vi "experiment control.vi"() -> ()   [LabVIEW 2012] (continued)
  T76 = cluster{"Wavemaster":cluster{"Serial Port":refnum<visa-resource-name>, "Wavelength":dbl, "Units":string, "VISA Name":refnum<visa-resource-name>, "Reading":bool, "Detected":bool}}
  T77 = cluster{"Header":cluster{"Element Names":string[], u8[]}, cluster{"Wavemaster":cluster{"Serial Port":refnum<visa-resource-name>, "Wavelength":dbl, "Units":string, "VISA Name":refnum<visa-resource-name>, "Reading":bool, "Detected":bool}}}
  T78 = cluster{"HP8341B":cluster{"GPIB Port":refnum<visa-resource-name>, "detected":bool, "rf":bool, "frequency":dbl, "stop frequency":dbl, "power":dbl, "sweep time":dbl, "Chirp":bool, "Pulse Modulate":bool, "Set frequency":dbl}}
  T79 = cluster{"Header":cluster{"Element Names":string[], u8[]}, cluster{"HP8341B":cluster{"GPIB Port":refnum<visa-resource-name>, "detected":bool, "rf":bool, "frequency":dbl, "stop frequency":dbl, "power":dbl, "sweep time":dbl, "Chirp":bool, "Pulse Modulate":bool, "Set frequency":dbl}}}
  T80 = cluster{"QuadDVM":cluster{"Serial Port":refnum<visa-resource-name>, "Quad DVM":dbl[][]}, "Magnetometer":cluster{"Active Boards":cluster{"Status":bool, "Board":string}[][], "USB ports":refnum<visa-resource-name>[], "Active Controllers":cluster{"Status":bool, "Number":dbl}[], "Measurements":cluster{"Bchip":dbl[][], "Status":dbl[], "Temperature":dbl, "Chip":dbl[], "Board":string, "Time":string}[]}, "Temperature Monitor":cluster{"measurements":cluster{"measurement":dbl, "location":string, "label":string}[], "last measurement time":string}}
  T81 = cluster{"Header":cluster{"Element Names":string[], u8[]}, cluster{"QuadDVM":cluster{"Serial Port":refnum<visa-resource-name>, "Quad DVM":dbl[][]}, "Magnetometer":cluster{"Active Boards":cluster{"Status":bool, "Board":string}[][], "USB ports":refnum<visa-resource-name>[], "Active Controllers":cluster{"Status":bool, "Number":dbl}[], "Measurements":cluster{"Bchip":dbl[][], "Status":dbl[], "Temperature":dbl, "Chip":dbl[], "Board":string, "Time":string}[]}, "Temperature Monitor":cluster{"measurements":cluster{"measurement":dbl, "location":string, "label":string}[], "last measurement time":string}}}
  T82 = cluster{"Frequency Counter":cluster{"GPIB Port":refnum<visa-resource-name>, "Frequency":dbl[]}}
  T83 = cluster{"Header":cluster{"Element Names":string[], u8[]}, cluster{"Frequency Counter":cluster{"GPIB Port":refnum<visa-resource-name>, "Frequency":dbl[]}}}
  T84 = cluster{"TDS5034B Oscilloscope":cluster{"GPIB Address":refnum<visa-resource-name>, "Detected":bool, "Channels":u16[], "Resolution":u16, "Frames":u16, "Trigger Position":dbl, "Trigger Level":dbl, "Measurements":cluster{"Type":string, "Value":dbl, "Source":string}[]}, "TDS2014 Oscilloscope":cluster{"GPIB Address":refnum<visa-resource-name>, "Detected":bool, "Channels":u16[], "Resolution":u16, "Frames":u16, "Trigger Position":dbl, "Trigger Level":dbl, "Measurements":cluster{"Type":string, "Value":dbl, "Source":string}[]}, "TDS5034B Data":cluster{"Y":dbl[], "t0":dbl, "dt":dbl}[], "TDS2014 Data":cluster{"Y":dbl[], "t0":dbl, "dt":dbl}[]}
  T85 = cluster{"Header":cluster{"Element Names":string[], u8[]}, cluster{"TDS5034B Oscilloscope":cluster{"GPIB Address":refnum<visa-resource-name>, "Detected":bool, "Channels":u16[], "Resolution":u16, "Frames":u16, "Trigger Position":dbl, "Trigger Level":dbl, "Measurements":cluster{"Type":string, "Value":dbl, "Source":string}[]}, "TDS2014 Oscilloscope":cluster{"GPIB Address":refnum<visa-resource-name>, "Detected":bool, "Channels":u16[], "Resolution":u16, "Frames":u16, "Trigger Position":dbl, "Trigger Level":dbl, "Measurements":cluster{"Type":string, "Value":dbl, "Source":string}[]}, "TDS5034B Data":cluster{"Y":dbl[], "t0":dbl, "dt":dbl}[], "TDS2014 Data":cluster{"Y":dbl[], "t0":dbl, "dt":dbl}[]}}
  T86 = cluster{"Trap Agilent":cluster{"USB":refnum<visa-resource-name>, "Amplitude":dbl, "Frequency":dbl, "Phase":dbl, "Upload":bool, "Output":bool}}
  T87 = cluster{"Header":cluster{"Element Names":string[], u8[]}, cluster{"Trap Agilent":cluster{"USB":refnum<visa-resource-name>, "Amplitude":dbl, "Frequency":dbl, "Phase":dbl, "Upload":bool, "Output":bool}}}
  T88 = cluster{"Jessica":T17, "Bertha":cluster{"wavelength":dbl, "locked":bool, "DIO64":string, "scan start":dbl, "scan end":dbl, "progress":u8, "scan step":dbl, "scan":bool, "setpoint":dbl, "wavelengths":dbl[]}, "Cora":cluster{"wavelength":dbl, "locked":bool, "DIO64":string, "scan start":dbl, "scan end":dbl, "progress":u8, "scan step":dbl, "scan":bool, "setpoint":dbl}, "Stella":cluster{"wavelength":dbl, "locked":bool, "lock tolerance":dbl, "setpoint":dbl, "scan start":dbl, "scan end":dbl, "progress":u8, "scan step":dbl, "scan":bool, "AI Channel":tag}, "Toptica":cluster{"wavelength":dbl, "locked":bool, "scan start":dbl, "scan end":dbl, "progress":u8, "scan step":dbl, "scan":bool, "AI Channel":tag}}
  T89 = cluster{"Header":cluster{"Element Names":string[], u8[]}, cluster{"Jessica":T17, "Bertha":cluster{"wavelength":dbl, "locked":bool, "DIO64":string, "scan start":dbl, "scan end":dbl, "progress":u8, "scan step":dbl, "scan":bool, "setpoint":dbl, "wavelengths":dbl[]}, "Cora":cluster{"wavelength":dbl, "locked":bool, "DIO64":string, "scan start":dbl, "scan end":dbl, "progress":u8, "scan step":dbl, "scan":bool, "setpoint":dbl}, "Stella":cluster{"wavelength":dbl, "locked":bool, "lock tolerance":dbl, "setpoint":dbl, "scan start":dbl, "scan end":dbl, "progress":u8, "scan step":dbl, "scan":bool, "AI Channel":tag}, "Toptica":cluster{"wavelength":dbl, "locked":bool, "scan start":dbl, "scan end":dbl, "progress":u8, "scan step":dbl, "scan":bool, "AI Channel":tag}}}
  T90 = cluster{"Header":cluster{"Element Names":string[], u8[]}, cluster{"Date":string, "Time":string}}
  T91 = cluster{"Switch Scan[0]":bool, "Switch Scan[1]":bool, "Switch Scan[2]":bool, "Switch Scan[3]":bool, "Switch Scan[4]":bool}
  T92 = cluster{"upper":dbl, "lower":dbl, "DurationUpper":dbl, "DurationLower":dbl, "Upper T":dbl, "Lower T":dbl}
  T93 = cluster{"Task":string, "begin time":dbl, "begin edge":bool, "begin reference":string, "end time":dbl, "end edge":bool, "end reference":string, "Chops":bool[]}
  T94 = cluster{"Down":cluster{"Frequency":dbl, "Phase":dbl, "Amplitude":dbl}[], "Up":cluster{"Frequency":dbl, "Phase":dbl, "Amplitude":dbl}[]}
  T95 = cluster{"Frequency":dbl, "Phase":dbl, "Amplitude":dbl}[]
  T96 = cluster{"Frequency":dbl, "Phase":dbl, "Duty Cycle":dbl, "Trigger":bool}[]
  T97 = cluster{"Frequency":dbl, "Phase":dbl, "Duty Cycle":dbl, "Trigger":bool}
  T98 = cluster{"variable":string, "scan string":string, "randomize":bool, "enable":bool}
  T99 = cluster{"Task":string, "Reference":string, "Begin":dbl, "Chops 2":bool[]}
  T100 = cluster{"Frequency":dbl, "Phase":dbl, "Amplitude":dbl}
  T101 = typedef "cw_template.ctl" = cluster{"wavelength":dbl, "name":string, "setpoint":dbl, "enable":bool, "lock":bool, "Priority":u8, "P":u8, "I":u8, "D":u8, "reset":bool, "analog channel":tag, "voltage":dbl, "exposure":u16, "range":dbl}
  T102 = typedef "pulse_template.ctl" = cluster{"wavelength":dbl, "name":string, "digital channel":tag}
  T103 = cluster{"Channel":string, "Name":string, "plot":bool}[]
  T104 = cluster{"system clock offset":bool, "system clock offset":bool, "open":bool, "open":bool, "multidevice sync mask":bool, "multidevice sync status":bool, "sync master enable":bool, "auto sync enable":bool, "open":bool, "open":bool, "open":bool, "open":bool, "all channel clear phase accumulator":bool, "all channel autoclear phase accumulator":bool, "all channel clear sweep accumulator":bool, "all channel autoclear sweep accumulator":bool}
  T105 = cluster{"Begin (ms)":dbl, "Begin (ms)":dbl, "DIO64 Line 1":bool[], "DIO64 Line 2":bool[], "DIO64 Line 3":bool[], "DIO64 Line 4":bool[]}
  T106 = cluster{"Begin (ms)":dbl, "Begin (ms)":dbl, "DIO64 Line 1":bool[], "DIO64 Line 2":bool[], "DIO64 Line 3":bool[], "DIO64 Line 4":bool[]}[]
  T107 = cluster{"Begin (ms)":dbl, "Begin (ms)":dbl, "DIO64 Line 4":bool[], "DIO64 Line 4":bool[], "DIO64 Line 4":bool[], "DIO64 Line 4":bool[]}
  T108 = cluster{"Begin (ms)":dbl, "Begin (ms)":dbl, "DIO64 Line 4":bool[], "DIO64 Line 4":bool[], "DIO64 Line 4":bool[], "DIO64 Line 4":bool[]}[]
  T109 = cluster{"Type":string, "Value":dbl, "Source":string}[]
  T110 = cluster{"Type":string, "Value":dbl, "Source":string}
  T111 = typedef "LVStringsAndValuesArrayTypeDef_U16.ctl" = cluster{"String":string, "Value":u16}[]
  T112 = typedef "LVRangeTypeDef.ctl" = cluster{"Minimum":dbl, "Maximum":dbl, "Increment":dbl, "Minor Increment":dbl, "Start":dbl}
  T113 = cluster{"start":dbl, "end":dbl, "ramp time":u8, "edge":bool}[]
  T114 = cluster{"Bchip":dbl[][], "Status":dbl[], "Temperature":dbl, "Chip":dbl[], "Board":string, "Time":string}[]
  T115 = cluster{"error":bool, "code":i32, "source":string}
  T116 = typedef "LVSelectionTypeDef.ctl" = cluster{"Selection Start":u32, "Selection End":u32}
  T117 = cluster{"32bit integer":i32, "32bit integer":u16}
  T118 = cluster{"Name":string, "DIO64 Line 1":bool[], "DIO64 Line 2":bool[], "DIO64 Line 3":bool[], "DIO64 Line 4":bool[]}
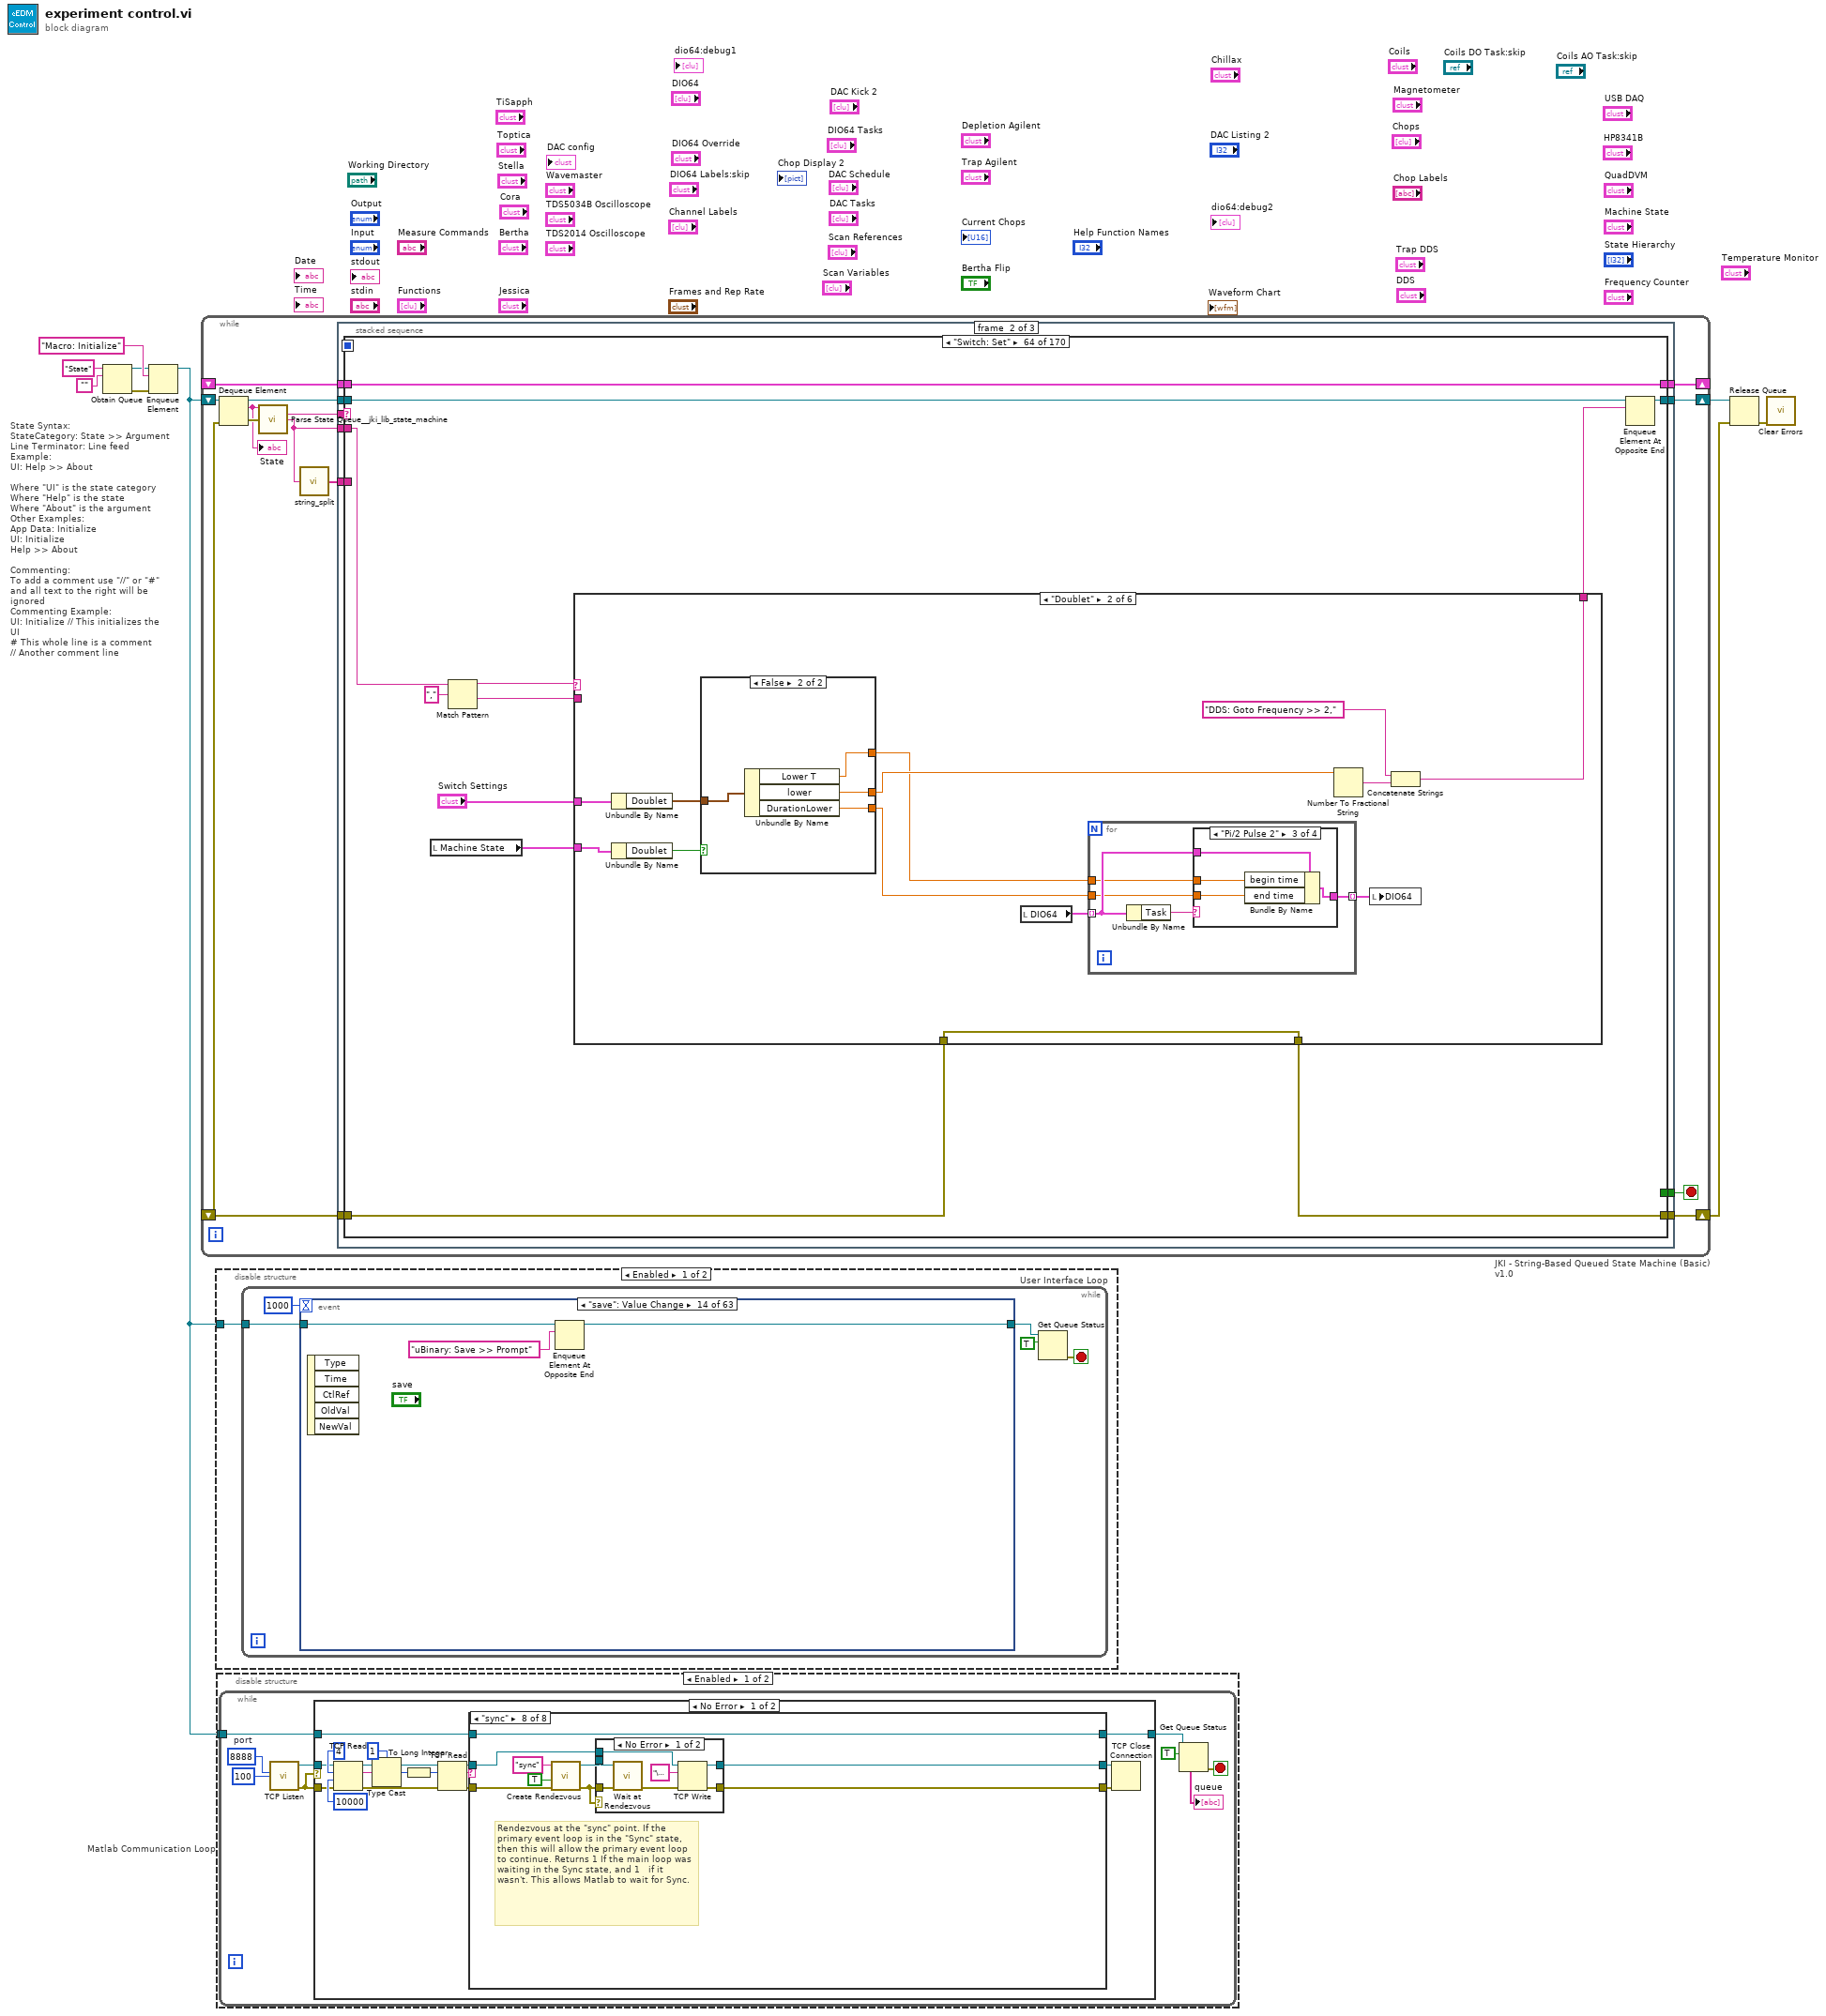
[diagram p0: block diagram]
diagram:
  # "State Syntax:\nStateCategory: State >> Argument\nLine Terminator: Line feed\nExample:\nUI: Help >> About\n\nWhere \"UI\" is the state category\nWhere \"Help\" is the state\nWhere \"About\" is the argument\nOther Examples:\nApp Data: Initialize\nUI: Initialize\nHelp >> About\n\nCommenting:\nTo add a comment use \"//\" or \"#\" and all text to the right will be ignored\nCommenting Example:\nUI: Initialize // This initializes the UI\n# This whole line is a comment\n// Another comment line"
  n1 = Obtain Queue(name (unnamed)="State", element data type="") -> (queue out=w5:refnum<queue>, error out=w6:errorcluster)  [unwired: 3 in, 1 out]
  n2 = Enqueue Element(queue=w5, element="Macro: Initialize", error in (no error)=w6) -> (queue out=w1:refnum<queue>)  [unwired: 1 in, 2 out]
  n3 = while "JKI - String-Based Queued State Machine (Basic) v1.0" {
    shift-right: [w18] -> _
    shift-left: _ -> [w21]
    shift-right: [w19] -> w3
    shift-left: _ -> [w15]
    shift-right: [w13] -> w4
    shift-left: w1 -> [w17]
    stop <- w20 stop-if-true
    n4 = Dequeue Element(queue=w17, error in (no error)=w15) -> (queue out=w16:refnum<queue>, element=w12:string, error out=w14:errorcluster)  [unwired: 1 in, 1 out]
    "State" <- w12
    n5 = call <vilib>:"Parse State Queue__jki_lib_state_machine.vi"("State Queue"=w12, "Error In (no error)"=w14) -> ("Current State"=w22:string, "Arguments"=w11:string)  [unwired: 11 in, 1 out]
    n6 = call "string_split.vi"("input"=w11) -> ("output"=w10:string[])
    n7 = stacked-sequence {
      seq-local: [w23 _ _] -> [_ _ w5598]
      tunnel: w22 -> [_ w33 w5600]
      tunnel: w11 -> [_ w32 _]
      tunnel: w21 -> [_ w31 w5599]
      tunnel: [_ w30 _] -> w20
      tunnel: [_ w29 _] -> w19
      tunnel: [_ w28 _] -> w18
      tunnel: w16 -> [_ w24 _]
      tunnel: w15 -> [_ w27 _]
      tunnel: [_ w26 _] -> w13
      tunnel: w10 -> [_ w25 _]
      frame #0 {
        n8 = Tick Count (ms)() -> (millisecond timer value=w23:u32)
      }
      frame #1 {
        n9 = case shown="\"Switch: Set\"" w33 {
          selector: w33 -> [_ _ _ w48 _ _ _ _ _ _ _ _ _ _ _ _ _ _ _ _ _ _ _ _ _ _ _ _ _ _ _ _ _ _ _ _ _ _ _ _ _ _ _ _ _ _ _ _ _ _ _ _ _ _ _ _ _ _ _ _ _ _ _ _ _ _ _ _ _ _ _ _ _ _ _ _ _ _ _ _ _ _ _ _ _ _ _ _ _ _ _ _ _ _ _ _ _ _ _ _ _ _ _ _ _ _ _ _ _ _ _ _ _ _ _ _ _ _ _ _ _ _ _ _ _ _ _ _ _ _ _ _ _ _ _ _ _ _ _ _ _ _ _ _ _ _ _ _ _ _ _ _ _ _ _ _ _ _ _ _ _ _ _ _ _ _ _ _ _ _]
          tunnel: w32 -> [_ _ _ _ _ _ _ _ _ _ _ _ w156 w165 _ _ _ _ _ _ _ _ _ _ _ _ _ _ w569 _ _ _ _ _ _ _ _ _ w719 w763 _ w925 _ w1144 w1785 _ w1944 _ w2139 w2149 _ _ _ w2218 _ _ _ w2443 w2461 _ _ _ _ w2540 w2664 _ _ w2735 w2897 w2912 _ w2935 w3121 w3238 _ _ _ w3375 w3380 _ _ _ _ _ _ _ _ _ w3526 _ w3650 _ w3758 _ _ w3808 w3821 w3860 w3925 w4004 w4091 w4125 w4161 w4307 w4322 _ _ _ _ _ _ _ _ _ _ _ _ w4618 w4684 _ _ _ _ _ w4896 w4969 _ _ _ _ _ _ _ _ _ _ _ _ _ _ _ _ _ _ w5232 _ _ _ _ _ _ _ _ _ _ _ _ _ _ _ w5413 _ _ _ _ _ _ _ _ _]
          tunnel: w31 -> [w40 w43 w45 w50 w60 w74 w87 w89 _ w113 w118 w132 w159 w167 w207 w228 w253 w274 w292 w312 w330 w371 w418 w494 w503 w523 w541 w558 w570 w593 w599 w605 w628 w654 w687 w697 w701 w712 w724 w773 w919 w921 w1116 w1140 w1787 w1933 w1942 w2130 w2140 w2150 w2156 w2182 w2202 w2223 w2292 w2418 w2433 w2449 w2467 w2481 w2489 w2510 w2517 w2541 w2662 w2704 w2720 w2738 w2898 w2913 w2930 w2936 w3122 w3239 w3362 w3369 w3371 w3376 w3381 w3389 w3403 w3411 w3429 w3447 w3466 w3482 w3489 w3498 w3527 w3573 w3653 w3732 w3761 w3783 w3785 w3809 w3822 w3857 w3926 w4005 w4092 w4126 w4159 w4308 w4323 w4331 w4345 w4351 w4364 w4437 w4495 w4501 w4508 w4533 w4555 w4568 w4578 w4619 w4685 w4756 w4769 w4781 w4786 w4888 w4891 w4970 w4982 w5002 w5014 w5046 w5059 w5065 w5067 w5110 w5118 w5132 w5141 w5143 w5155 w5178 w5185 w5191 w5193 w5213 w5235 w5244 w5257 w5266 w5268 w5283 w5305 w5311 w5313 w5327 w5334 w5340 w5365 w5371 w5373 w5389 w5416 w5452 w5454 w5463 w5480 w5498 w5516 w5538 w5556 w5576]
          tunnel: [w36 w41 w46 w52 w66 w68 w86 w90 w110 w114 w119 w131 w157 w168 w195 w227 w252 w273 w291 w310 w329 w372 w417 w495 w496 w518 w528 w559 w561 w594 w595 w600 w629 w658 w688 w689 w702 w703 w715 w766 w920 w926 w1118 w1142 w1788 w1934 w1946 w2131 w2141 w2151 w2158 w2183 w2189 w2221 w2291 w2405 w2434 w2445 w2463 w2482 w2490 w2512 w2518 w2538 w2663 w2705 w2721 w2736 w2899 w2914 w2931 w2933 w3119 w3236 w3355 w3366 w3372 w3377 w3382 w3390 w3401 w3409 w3427 w3445 w3464 w3480 w3490 w3496 w3524 w3571 w3651 w3730 w3759 w3781 w3786 w3806 w3819 w3858 w3923 w4002 w4089 w4123 w4160 w4305 w4320 w4332 w4343 w4349 w4362 w4435 w4493 w4499 w4506 w4531 w4556 w4566 w4577 w4616 w4682 w4757 w4759 w4776 w4782 w4889 w4895 w4968 w4977 w5003 w5012 w5015 w5057 w5063 w5068 w5073 w5111 w5123 w5134 w5144 w5153 w5176 w5183 w5189 w5194 w5211 w5233 w5242 w5255 w5264 w5269 w5274 w5292 w5309 w5314 w5326 w5335 w5338 w5362 w5368 w5374 w5387 w5414 w5450 w5455 w5456 w5478 w5496 w5514 w5536 w5554 w5574] -> w29
          tunnel: w27 -> [w37 w41 w46 w51 w66 w69 w86 w90 w110 w115 w119 w131 w158 w169 w192 w226 w251 w273 w291 w311 w329 w351 w426 w495 w497 w517 w529 w559 w562 w594 w596 w601 w631 w659 w688 w690 w702 w704 w716 w767 w920 w927 w1115 w1143 w1789 w1934 w1943 w2131 w2141 w2151 w2170 w2183 w2192 w2222 w2291 w2406 w2434 w2446 w2464 w2482 w2490 w2512 w2518 w2539 w2663 w2705 w2721 w2737 w2899 w2914 w2931 w2934 w3120 w3237 w3354 w3365 w3372 w3377 w3382 w3390 w3402 w3410 w3428 w3446 w3465 w3481 w3490 w3497 w3525 w3572 w3652 w3731 w3760 w3782 w3786 w3807 w3820 w3859 w3924 w4003 w4090 w4124 w4160 w4306 w4321 w4332 w4344 w4350 w4363 w4436 w4494 w4500 w4507 w4532 w4556 w4567 w4576 w4617 w4683 w4757 w4765 w4777 w4783 w4889 w4894 w4968 w4978 w5003 w5013 w5045 w5058 w5064 w5068 w5109 w5114 w5129 w5137 w5144 w5154 w5177 w5184 w5190 w5194 w5212 w5234 w5243 w5256 w5265 w5269 w5275 w5293 w5310 w5314 w5325 w5335 w5337 w5363 w5369 w5374 w5388 w5415 w5451 w5455 w5457 w5479 w5497 w5515 w5537 w5555 w5575]
          tunnel: [w34 w42 w44 w47 w57 w72 w84 w88 w95 w112 w117 w125 w155 w164 w206 w225 w250 w272 w290 w302 w318 w369 w442 w493 w498 w519 w527 w557 w560 w591 w598 w602 w630 w657 w685 w696 w698 w706 w718 w769 w918 w922 w1117 w1135 w1782 w1930 w1936 w2117 w2132 w2142 w2159 w2184 w2203 w2224 w2293 w2419 w2431 w2447 w2465 w2480 w2483 w2499 w2514 w2532 w2646 w2695 w2719 w2722 w2890 w2911 w2929 w2932 w3118 w3235 w3361 w3368 w3370 w3373 w3379 w3388 w3392 w3404 w3422 w3440 w3459 w3476 w3488 w3491 w3523 w3570 w3633 w3714 w3733 w3778 w3784 w3788 w3815 w3855 w3922 w4001 w4088 w4122 w4158 w4304 w4319 w4330 w4342 w4346 w4359 w4434 w4492 w4498 w4503 w4530 w4554 w4565 w4575 w4615 w4664 w4755 w4760 w4779 w4785 w4887 w4893 w4957 w4986 w5001 w5011 w5044 w5056 w5060 w5066 w5108 w5117 w5131 w5140 w5142 w5152 w5175 w5182 w5186 w5192 w5195 w5231 w5241 w5254 w5258 w5267 w5282 w5302 w5308 w5312 w5324 w5333 w5339 w5364 w5370 w5372 w5375 w5406 w5449 w5453 w5458 w5475 w5493 w5511 w5533 w5553 w5569] -> w26
          tunnel: [_ _ _ _ _ _ TRUE _ _ _ _ _ _ _ _ _ _ _ _ _ _ _ _ _ _ _ _ _ _ _ _ _ _ _ _ _ _ _ _ _ _ _ _ _ _ _ _ _ _ _ _ _ _ _ _ _ _ _ _ _ _ _ _ _ _ _ _ _ _ _ _ _ _ _ _ _ _ _ _ _ _ _ _ _ _ _ _ _ _ _ _ _ _ _ _ _ _ _ _ _ _ _ _ _ _ _ _ _ _ _ _ _ _ _ _ _ _ _ _ _ _ _ _ _ _ _ _ _ _ _ _ _ _ _ _ _ _ _ _ _ _ _ _ _ _ _ _ _ _ _ _ _ _ _ _ _ _ _ _ _ _ _ _ _ _ _ _ _ _ _] -> w30
          tunnel: [w40 w43 w45 w50 w67 w74 w87 w89 w111 w113 w118 w132 w159 w167 w207 w228 w253 w274 w292 w312 w330 w370 w418 w494 w503 w523 w541 w558 w570 w593 w599 w605 w633 w653 w687 w697 w700 w712 w724 w773 w919 w924 w1116 w1141 w1786 w1935 w1945 w2130 w2140 w2150 w2155 w2182 w2202 w2223 w2292 w2418 w2433 w2449 w2467 w2481 w2488 w2511 w2517 w2541 w2661 w2703 w2720 w2738 w2898 w2913 w2930 w2936 w3122 w3239 w3362 w3369 w3371 w3376 w3381 w3389 w3403 w3411 w3429 w3447 w3466 w3482 w3489 w3498 w3527 w3573 w3653 w3732 w3761 w3783 w3785 w3809 w3822 w3856 w3926 w4005 w4092 w4126 w4159 w4308 w4323 w4331 w4345 w4351 w4364 w4437 w4495 w4501 w4508 w4533 w4555 w4568 w4578 w4619 w4685 w4756 w4769 w4781 w4786 w4888 w4890 w4970 w4981 w5002 w5014 w5046 w5059 w5065 w5067 w5110 w5118 w5132 w5141 w5143 w5155 w5178 w5185 w5191 w5193 w5213 w5235 w5244 w5257 w5266 w5268 w5283 w5305 w5311 w5313 w5327 w5334 w5340 w5365 w5371 w5373 w5389 w5416 w5452 w5454 w5463 w5480 w5498 w5516 w5538 w5556 w5576] -> w28
          tunnel: w25 -> [_ _ _ _ _ _ _ _ _ _ _ _ _ _ _ _ _ _ _ _ _ _ _ _ _ _ _ _ _ _ _ _ _ _ w684 _ _ _ _ _ w883 _ w1108 _ _ _ _ w2114 _ _ w2153 _ _ w2216 _ _ _ _ _ _ _ _ _ _ _ _ _ _ _ _ _ _ _ _ _ _ _ _ _ _ _ _ _ _ _ _ _ _ _ _ _ _ _ _ _ _ _ _ _ _ _ _ _ _ _ _ _ _ _ _ _ _ _ _ _ _ _ _ _ _ _ _ w4784 _ _ _ _ _ _ _ _ _ _ _ _ _ _ _ _ _ _ _ _ _ _ _ _ _ _ _ _ _ _ _ _ _ _ _ _ _ _ _ _ _ _ _ _ _ _ _]
          tunnel: w24 -> [w35 w42 w44 w47 w57 w71 w84 w88 w95 w112 w117 w125 w155 w164 w206 w225 w250 w272 w290 w302 w318 w369 w442 w493 w498 w520 w531 w557 w560 w591 w597 w604 w632 w660 w685 w696 w698 w706 w718 w769 w918 w922 w1117 w1135 w1782 w1930 w1936 w2117 w2132 w2142 w2159 w2184 w2203 w2224 w2293 w2419 w2432 w2448 w2466 w2480 w2483 w2498 w2514 w2530 w2645 w2695 w2719 w2722 w2890 w2911 w2929 w2932 w3118 w3235 w3361 w3368 w3370 w3373 w3379 w3388 w3392 w3404 w3422 w3440 w3459 w3476 w3488 w3491 w3523 w3570 w3633 w3714 w3733 w3778 w3784 w3788 w3815 w3855 w3922 w4001 w4088 w4122 w4158 w4304 w4319 w4330 w4342 w4346 w4359 w4434 w4492 w4498 w4503 w4530 w4554 w4565 w4575 w4615 w4664 w4755 w4761 w4779 w4785 w4887 w4893 w4957 w4986 w5001 w5011 w5044 w5056 w5060 w5066 w5108 w5117 w5131 w5140 w5142 w5152 w5175 w5182 w5186 w5192 w5195 w5231 w5241 w5254 w5258 w5267 w5282 w5302 w5308 w5312 w5324 w5333 w5339 w5364 w5370 w5372 w5375 w5406 w5449 w5453 w5459 w5475 w5493 w5511 w5533 w5553 w5569]
          frame "Idle" {
            # "executes when the state queue is empty"
            n10 = call "string_to_array.vi"("string"="Temperature: Read\nMacro: Read Wavelengths") -> ("array"=w38:string[])
            n11 = call "queue_array_front.vi"("error in"=w37, "array"=w38, "queue in"=w35) -> ("error out"=w36:errorcluster, "queue out"=w34:refnum<queue>)  [unwired: 7 in]
          }
          frame "" {
            # "executes when the state queue is empty"
          }
          frame "---------- Core ----------" {
            # "Do not put any code in this frame.\n(it is a separator no-op)"
          }
          frame Default {
            w55 = 42 items=["No error", "Argument error", "Memory is full", "Out of zone", "End of file", "File already open", "Generic file I/O error", "File not found", "File permission error", "Disk is full", "Duplicate path", "Too many files open", "System feature not enabled", "Resource file not found", "Cannot add resource", "Resource not found", "Image not found", "Image memory error", "Pen does not exist", "Config type invalid", "Config token not found", "Config parse error", "Config memory error", "Bad external code format", "Bad external code offset", "External code not present", "Null window", "Destroy window error", "Null menu", "Print aborted", "Bad print record", "Print driver error", "Windows error during printing", "Memory error during printing", "Print dialog error", "Generic print error", "Invalid device refnum", "Device not found", "Device parameter error", "Device unit error", "Cannot open device", "Device call aborted", "Generic error", "Cancelled by user", "Object ID too low", "Object ID too high", "Object not in heap", "Unknown heap", "Unknown object (invalid DefProc)", "Unknown object (DefProc not in table)", "Message out of range", "Invalid (null) method", "Unknown message", "Manager call not supported", "Bad address", "Network operation in progress", "Network operation timed out", "Connection is busy", "Network attribute not supported", "Network error", "Address in use", "System out of memory", "Connection aborted", "Connection refused", "Not connected", "Already connected", "Connection closed", "Initialization error (interapplication manager)", "Bad occurrence", "Wait on unbound occurrence handler", "Occurrence queue overflow", "Datalog type conflict", "Unused", "Unrecognized type (interapplication manager)", "Memory corrupt", "Failed to make temporary DLL", "Old CIN version", "Drag socket not found", "Failed to load drop-object", "Failed to register OLE object", "Failed to release OLE object", "Format specifier type mismatch", "Unknown format specifier", "Too few format specifiers", "Too many format specifiers", "Scan failed", "Newer CIN version", "Error converting to variant", "Runtime menu error", "Password tampered", "Variant attribute not found", "Incompatible variant data type", "Event data is not available", "Event Store is not present", "Occurrence is not found", "Event Queue is not created", "Event info is not available", "Refnum passed is NULL", "Error retrieving Class GUID", "Error retrieving CoClass GUID", "Error retrieving TypeLib GUID.", "Bad built application magic bytes.", "Specific driver is different from the specific driver associated with the Logical Name.", "There is no session opened to the class driver.", "Max Error", "MAX - Error with config objects", "MAX - Error loading configuration", "MAX - Group not supported"]
            # "Current State"
            # "Do not delete, rename, or modify this frame.\n(this is used to capture unhandled states and typos)"
            # "Handle mistyped state name (developer tool)"
            n12 = Format Into String(format string="Software Exception: Unhandled State \"%s\"." ("message"), error in=w51, w48) -> (resulting string=w54:string, error out=w53:errorcluster)  [unwired: 1 in]
            n13 = call <vilib>:"Error Cluster From Error Code.vi"("show call chain? (False)"=TRUE, "error in (no error)"=w53, "error message (\"\")"=w54, "error code (0)"=w55) -> ("error out"=w52:errorcluster)  [unwired: 5 in]
          }
          frame "Initialize Core Data" {
            # "Do not delete, rename, or modify this frame.\n(this is used to determine panel behavior on exit)"
            # "originally closed?"
            # "exe?"
            # "If panel starts closed or is an EXE, then close it when we exit"
            n14 = property class="VI"() -> ("Front Panel.Open"=w65:bool)  [unwired: 2 in, 2 out]
            n15 = property class="App"() -> ("App.Kind"=w64:T38)  [unwired: 2 in, 2 out]
            n16 = control-ref of="Current VI Reference"() -> (w58:refnum<vi>)
            n17 = Not(x=w65) -> (.not. x?=w62:bool)
            n18 = Equal?(x=w64, y=T38."Run Time System" ("Application:Kind")) -> (x = y?=w61:bool)
            n19 = Or(x=w62, y=w61) -> (x .or. y?=w59:bool)
            n20 = Bundle By Name(cluster=w60, "Core.Current VI Reference"=w58, "Core.Close Panel on Exit?"=w59) -> (w67:T52)
          }
          frame "Error Handler" {
            # "Handle any errors here.\nYou can also output any states to clean-up after errors occur"
            n21 = call <vilib>:"Clear Errors.vi"("error in (no error)"=w69) -> ("error out"=w68:errorcluster)  [unwired: 6 in]
            n22 = Unbundle By Name(w69) -> ("source"=w73:string)
            n23 = stacked-sequence {
              tunnel: w73 -> [w79 _]
              frame #0 {
                n24 = local read "stdout"() -> (w81:string)
                n25 = Get Date/Time String() -> (date string=w76:string, time string=w77:string)  [unwired: 3 in]
                n26 = Concatenate Strings(w81, "\r\n", w76, " " ("string"), w77, ": " ("string"), w79) -> (w82:string)
                n27 = local write "stdout"(w82) -> ()
              }
              frame #1 {
                n28 = property on="stdout" class="Str"("Text.Scroll Position"=u32 4294967295) -> ()  [unwired: 2 in, 2 out]
              }
            }
            n29 = Enqueue Element At Opposite End(queue=w71, element="/* Post Error States") -> (queue out=w72:refnum<queue>)  [unwired: 2 in, 2 out]
          }
          frame "Exit" {
            # "Do not put any code in this frame.\n(No errors that occur here will be handled.)"
          }
          frame "---------- Data ----------" {
            # "Do not put any code in this frame.\n(It is a separator no-op. You can make a copy of this frame to create a new Data frame)"
          }
          frame "Data: Initialize" {
            w91 = T7 {"loaded"=FALSE, "output 1"="", "clock 1"="", "output 2"="", "clock 2"=""}  # dac state
            w92 = refnum<k5> refnum  # img mcp tcp
            w93 = u32 0  # Idle Timer
            w94 = string[] []  # Paused Queue
            w96 = u32 0  # Block Index
            w97 = path ""  # Block Prefix
            w98 = FALSE  # Paused
            w99 = bool[][] []  # Switch Scan
            w100 = 0  # Switch Scan Index
            w101 = cluster{"Y":dbl[], "t0":dbl, "dt":dbl}[] []  # TDS2014 Data
            w102 = cluster{"Y":dbl[], "t0":dbl, "dt":dbl}[] []  # TDS5034B Data
            w103 = u32 0  # Scan Index
            w104 = path ""  # Scan Prefix
            w105 = ""  # Do Loop Contents
            w106 = u32 0  # Time
            w107 = string[] []  # Command Names
            w108 = string[] []  # Command History
            w109 = T53 {"Current VI Reference"=refnum, "Close Panel on Exit?"=FALSE}  # Core
            # "These are for the CLI history\nand tab completion"
            # "do not delete - used by framework"
            # "Data names and types of shift register data are defined by this bundle."
            # "Initialize the shift-register data, here.\n(data names are defined by what you wire into the bundle function)"
            n30 = Bundle("Core"=w109, "Command History"=w108, "Command Names"=w107, "Time"=w106, "Do Loop Contents"=w105, "Scan Prefix"=w104, "Scan Index"=w103, "Switch Scan Index"=w100, "Switch Scan"=w99, "Paused"=w98, "Paused Queue"=w94, "Block Prefix"=w97, "dac state"=w91, "Block Index"=w96, "Idle Timer"=w93, "img mcp tcp"=w92, "TDS5034B Data"=w102, "TDS2014 Data"=w101) -> (w111:T52)  [unwired: 1 in]
          }
          frame "Data: Cleanup" {
            # "Cleanup any data and references, here.\n(this is called automatically, by the Macro: Exit)"
            n31 = Unbundle By Name(w113) -> ("Core.Current VI Reference"=w116:refnum<vi>)
            n32 = Close Reference(reference=w116, error in (no error)=w115) -> (error out=w114:errorcluster)
          }
          frame "---------- UI ----------" {
            # "Do not put any code in this frame.\n(It is a separator no-op. You can make a copy of this frame to create a new UI frame)"
          }
          frame "UI: Initialize" {
            w130 = FALSE ("stop")
            # "Initialize the User Interface, here.\n(this is called automatically, by the Macro: Init)"
            n33 = local write "pause:skip"(FALSE ("Pause")) -> ()
            n34 = local write "stop"(w130) -> ()
            n35 = local write "Test"(w130) -> ()
            n36 = local read "Channel Labels"() -> (w127:T10)
            n37 = property on="test" class="Bool (strict)"("DisabledEnum"=T39."Disabled and Grayed Out" ("Disabled")) -> ()  [unwired: 2 in, 2 out]
            n38 = for {
              tunnel: w127 -> [w142] mode=indexing
              tunnel: [w140] -> w126 mode=indexing
              i -> [w141]
              n39 = for {
                tunnel: w142 -> [w145] mode=indexing
                tunnel: w141 -> [w148]
                tunnel: [w143] -> w140 mode=indexing
                i -> [w154]
                n40 = Add(x=65, y=w154) -> (x+y=w150:i32)
                n41 = To Unsigned Byte Integer(number=w150) -> (unsigned 8bit integer=w149:u8)
                n42 = Format Value(format string="%02d:", value (0)=w148) -> (output string=w147:string)  [unwired: 1 in]
                n43 = Type Cast(type="" ("*(type *) &x"), x=w149) -> (*(type *) &x=w151:string)
                n44 = Concatenate Strings(w151, w147) -> (w144:string)
                n45 = Bundle By Name(cluster=w145, "Channel"=w144) -> (w143:T54)
              }
            }
            n46 = property on="Input" class="TabCtl (strict)"() -> ("Pages"=w122:refnum<vi>[])  [unwired: 2 in, 2 out]
            n47 = property on="Output" class="TabCtl (strict)"() -> ("Pages"=w121:refnum<vi>[])  [unwired: 2 in, 2 out]
            n48 = Build Array (concatenate)(w122, w121) -> (w120:refnum<vi>[])
            n49 = for {
              tunnel: w120 -> [w139] mode=indexing
              n50 = property class="Page"(reference=w139) -> (reference out=w136:refnum<vi>, error out=w135:errorcluster, "PageLabel"=w138:string)  [unwired: 1 in]
              n51 = Match Pattern(string=w138, regular expression="^hidden:") -> (offset past match=w134:i32)  [unwired: 1 in, 3 out]
              n52 = Less Than 0?(x=w134) -> (x < 0?=w133:bool)
              n53 = property class="Page"(reference=w136, error in=w135, "PageVis"=w133) -> ()  [unwired: 2 out]
            }
            n54 = local write "Channel Labels"(w126) -> ()
            n55 = property on="img mcp" class="IntGraph (strict)"("ZScale.MarkerVals[]"=cluster{dbl, u32}[] [{0.0, 0}, {255.0, 16448250}] ("Z Scale.Marker Values[]")) -> ()  [unwired: 2 in, 2 out]
            n56 = property on="State Hierarchy" class="LstBox (strict)"("Value"=i32[] [] ("State Hierarchy")) -> ()  [unwired: 2 in, 2 out]
          }
          frame "UI: Cursor Set" {
            # "Argument"
            # "Set and Unset Cursor Busy.\n(Usage: \"UI: Cursor Set >> Busy|Idle\")"
            n57 = case shown="\"Busy\"" w156 {
              tunnel: w158 -> [w161 w163]
              tunnel: [w160 w162] -> w157
              frame "Idle", Default {
                n58 = call <vilib>:"Unset Busy.vi"("error in (no error)"=w161) -> ("error out"=w160:errorcluster)  [unwired: 10 in]
              }
              frame "Busy" {
                n59 = call <vilib>:"Set Busy.vi"("error in (no error)"=w163) -> ("error out"=w162:errorcluster)  [unwired: 9 in, 1 out]
              }
            }
          }
          frame "UI: Front Panel State" {
            # "Argument"
            # "Set Front Panel Open or Closed\n(Usage: \"UI: Front Panel State >> Open|Close\")"
            n60 = Unbundle By Name(w167) -> ("Core.Current VI Reference"=w166:refnum<vi>)
            n61 = case shown="\"Open\", Default" w165 {
              tunnel: w169 -> [w173 w186]
              tunnel: [w175 w187] -> w168
              tunnel: w166 -> [w174 w184]
              frame "Open", Default {
                n62 = property class="VI"(reference=w174, error in=w173) -> (reference out=w171:refnum<vi>, error out=w172:errorcluster, "Front Panel.Open"=w170:bool)
                n63 = case shown="True" w170 {
                  tunnel: [w178 w181] -> w175
                  tunnel: w172 -> [w177 w181]
                  tunnel: w171 -> [w176 _]
                  frame False {
                    n64 = invoke class="VI" method="FP.Open"(reference=w176, error in=w177, "Activate"=TRUE, "State"=T40."Standard") -> (error out=w178:errorcluster)  [unwired: 1 in, 4 out]
                  }
                  frame True {
                  }
                }
              }
              frame "Close" {
                n65 = property class="VI"(reference=w184, error in=w186) -> (reference out=w183:refnum<vi>, error out=w185:errorcluster, "Front Panel.Open"=w182:bool)
                n66 = case shown="True" w182 {
                  tunnel: [w188 w191] -> w187
                  tunnel: w185 -> [w188 w190]
                  tunnel: w183 -> [_ w189]
                  frame False {
                  }
                  frame True {
                    n67 = invoke class="VI" method="FP.Close"(reference=w189, error in=w190) -> (error out=w191:errorcluster)  [unwired: 1 in, 2 out]
                  }
                }
              }
            }
          }
          frame "UI: DIO64 Update Control" {
            w201 = "<SELF>"
            w204 = "T0"
            # "This is added to the queue whenever the DIO64 Tasks is updated. It calculates the cumulative time"
            n68 = local read "DIO64 Tasks"() -> (w205:T4)
            n69 = for {
              tunnel: w205 -> [w210] mode=indexing
              tunnel: [w209] -> w202 mode=indexing
              n70 = Unbundle By Name(w210) -> ("Name"=w208:string)
              n71 = Bundle("Name"=w208, "Name"=w208) -> (w209:cluster{"Name":string, "Name":string})  [unwired: 1 in]
            }
            n72 = Bundle(w204, w204) -> (w203:cluster{string, string})  [unwired: 1 in]
            n73 = Bundle(w201, w201) -> (w200:cluster{string, string})  [unwired: 1 in]
            n74 = Build Array (concatenate)(w203, w202) -> (w199:cluster{"Name":string, "Name":string}[])
            n75 = Build Array (concatenate)(w200, w199) -> (w198:cluster{"Name":string, "Name":string}[])
            n76 = property on="Task" class="CmbBox"(error in=w192, "Strings And Values[]"=w202) -> (error out=w193:errorcluster)  [unwired: 1 in, 1 out]
            n77 = property on="begin reference" class="CmbBox"(error in=w192, "Strings And Values[]"=w199) -> (error out=w194:errorcluster)  [unwired: 1 in, 1 out]
            n78 = property on="end reference" class="CmbBox"(error in=w192, "Strings And Values[]"=w198) -> (error out=w196:errorcluster)  [unwired: 1 in, 1 out]
            n79 = Merge Errors(w193, w194, w196) -> (w195:errorcluster)
            n80 = Enqueue Element At Opposite End(queue=w206, element="UI: Update Scan References") -> ()  [unwired: 2 in, 3 out]
          }
          frame "UI: Update Scan References" {
            w215 = string[] ["Lisa Wavelength", "Jessica Wavelength", "DDG CHA Delay", "DDG CHB Delay", "DDG CHC Delay", "DDG CHD Delay", "DDG CHE Delay", "DDG CHF Delay", "DDG CHG Delay", "DDG CHH Delay", "DDS Channel 1", "DDS Channel 2", "DDS Channel 3", "DDS Channel 4", "Microwave Begin", "Microwave End", "Microwave Power", "Doublet Upper T", "Doublet Lower T", "Trap DDS Frequency", "Brot"]
            # "This is added to the queue whenever the DIO64 Tasks is updated. It calculates the cumulative time"
            n81 = local read "DIO64 Tasks"() -> (w224:T4)
            n82 = local read "DAC Tasks"() -> (w218:T8)
            n83 = for {
              tunnel: w224 -> [w245] mode=indexing
              tunnel: [w243] -> w223 mode=indexing
              tunnel: [w241] -> w222 mode=indexing
              tunnel: [w237] -> w217 mode=indexing
              tunnel: [w236] -> w216 mode=indexing
              n84 = Unbundle By Name(w245) -> ("Name"=w240:string)
              n85 = Concatenate Strings(w240, " Begin" ("string")) -> (w243:string)
